vi "_027.vi"() -> ()   [LabVIEW 2024]
panel:
  in  "stop":bool
  out "Green":bool
  out "Yellow":bool
  out "Red":bool
  # "Local Variable :"
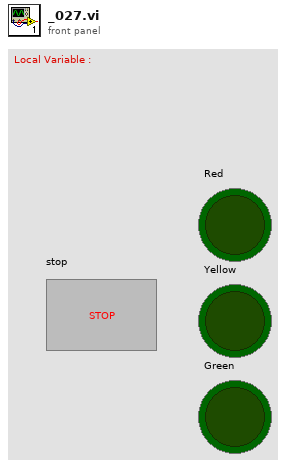
[diagram p1: front panel]
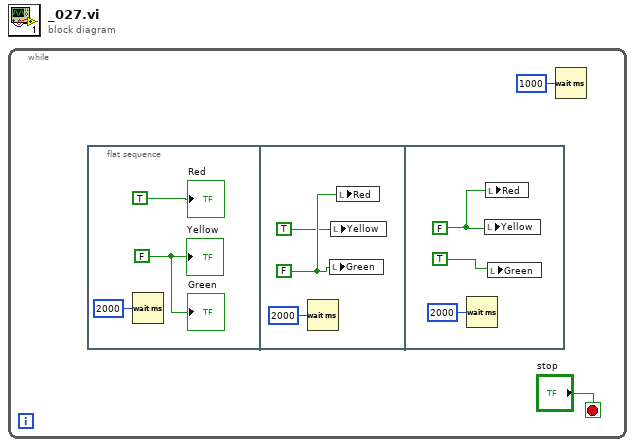
[diagram p0: block diagram]
diagram:
  n1 = while {
    stop <- "stop" stop-if-true
    n2 = flat-sequence {
      frame #0 {
        w4 = FALSE
        n3 = Wait (ms)(milliseconds to wait=u32 2000) -> ()  [unwired: 1 out]
        "Red" <- TRUE
        "Yellow" <- w4
        "Green" <- w4
      }
      frame #1 {
        w8 = FALSE
        n4 = Wait (ms)(milliseconds to wait=u32 2000) -> ()  [unwired: 1 out]
        n5 = local write "Green"(w8) -> ()
        n6 = local write "Yellow"(TRUE) -> ()
        n7 = local write "Red"(w8) -> ()
      }
      frame #2 {
        w10 = FALSE
        n8 = Wait (ms)(milliseconds to wait=u32 2000) -> ()  [unwired: 1 out]
        n9 = local write "Yellow"(w10) -> ()
        n10 = local write "Red"(w10) -> ()
        n11 = local write "Green"(TRUE) -> ()
      }
    }
    n12 = Wait (ms)(milliseconds to wait=u32 1000) -> ()  [unwired: 1 out]
  }
